vi "Actor Core.vi"(8 "error in":cluster{"状态":bool, "代码":i32, "源":string} caption="错误输入", 11 "JOY in":refnum<class "JoyStick.lvclass">) -> (0 "error out":cluster{"状态":bool, "代码":i32, "源":string} caption="错误输出", 3 "操作者输出":refnum<class "Actor.lvclass">)   [LabVIEW 2014, in "JoyStick.lvlib" / "JoyStick.lvclass"]
doc: "Actor Core.vi包含操作者的主要消息处理循环。操作者通常位于该循环中，在各种消息到达时对消息进行处理。如Do.vi消息返回任何错误，该循环将停止运行，错误代码43将被作为“无错误停止”的标准信号发送给调用方。如需更改上述行为，可在子孙类的Handle Error.vi中对该部分逻辑进行重写。"
uses:
  JoyStick.lvclass
  <vilib>/ActorFramework/Actor/Actor.lvclass
  <vilib>/MakerHub/Xbox-One-Controller/Private/Type Defs/Indicators/All Buttons Visual.ctl
  <vilib>/MakerHub/Xbox-One-Controller/Private/Type Defs/Indicators/A.ctl
  <vilib>/MakerHub/Xbox-One-Controller/Private/Type Defs/Indicators/B.ctl
  <vilib>/MakerHub/Xbox-One-Controller/Private/Type Defs/Indicators/X.ctl
  <vilib>/MakerHub/Xbox-One-Controller/Private/Type Defs/Indicators/Y.ctl
  <vilib>/MakerHub/Xbox-One-Controller/Private/Type Defs/Indicators/Left Bumper.ctl
  <vilib>/MakerHub/Xbox-One-Controller/Private/Type Defs/Indicators/Right Bumper.ctl
  <vilib>/MakerHub/Xbox-One-Controller/Private/Type Defs/Indicators/View.ctl
  <vilib>/MakerHub/Xbox-One-Controller/Private/Type Defs/Indicators/Menu.ctl
  <vilib>/MakerHub/Xbox-One-Controller/Private/Type Defs/Indicators/Thumbstick.ctl
  <vilib>/MakerHub/Xbox-One-Controller/Private/Type Defs/Indicators/All Axis Data.ctl
  <vilib>/MakerHub/Xbox-One-Controller/Private/Type Defs/Indicators/DPad Enum.ctl
  <vilib>/ActorFramework/Actor/Actor.lvclass/Actor.ctl
  JoyStick.lvclass/JoyStick.ctl
  <vilib>/ActorFramework/Message Enqueuer/Message Enqueuer.lvclass/Message Enqueuer.ctl
  <vilib>/ActorFramework/Message Enqueuer/Enqueue.vi
  <vilib>/MakerHub/Xbox-One-Controller/Public/Open First Controller.vi
  <vilib>/ActorFramework/Message Priority Queue/Priority Enqueue.vi
  Wrapper_lib/zsActor/ActorWrapper.lvclass
  <vilib>/MakerHub/Xbox-One-Controller/LMH-Xbox-One-Controller.lvlib
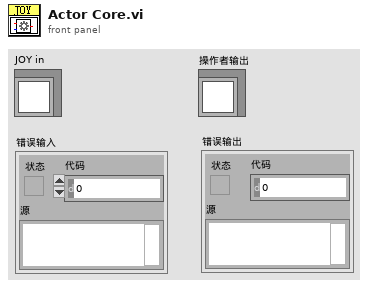
[diagram p1: front panel]
types:
  T1 = typedef "LMH-Xbox-One-Controller.lvlib/All Buttons Visual.ctl" = cluster{"A":T2, "B":T3, "X":T4, "Y":T5, "Left Bumper":T6, "Right Bumper":T7, "View Button":T8, "Menu Button":T9, "Left Stick":T10, "Right Stick":T10}
  T2 = typedef "LMH-Xbox-One-Controller.lvlib/A.ctl" = bool
  T3 = typedef "LMH-Xbox-One-Controller.lvlib/B.ctl" = bool
  T4 = typedef "LMH-Xbox-One-Controller.lvlib/X.ctl" = bool
  T5 = typedef "LMH-Xbox-One-Controller.lvlib/Y.ctl" = bool
  T6 = typedef "LMH-Xbox-One-Controller.lvlib/Left Bumper.ctl" = bool
  T7 = typedef "LMH-Xbox-One-Controller.lvlib/Right Bumper.ctl" = bool
  T8 = typedef "LMH-Xbox-One-Controller.lvlib/View.ctl" = bool
  T9 = typedef "LMH-Xbox-One-Controller.lvlib/Menu.ctl" = bool
  T10 = typedef "LMH-Xbox-One-Controller.lvlib/Thumbstick.ctl" = bool
  T11 = typedef "LMH-Xbox-One-Controller.lvlib/All Axis Data.ctl" = cluster{"Left Stick":cluster{"X Axis":i32, "Y Axis":i32}, "Right Stick":cluster{"X Axis":i32, "Y Axis":i32}, "Triggers":i32, "D-Pad":T12}
  T12 = typedef "LMH-Xbox-One-Controller.lvlib/DPad Enum.ctl" = enum16{"Idle", "Up", "Up / Right", "Right", "Down / Right", "Down", "Down / Left", "Left", "Up / Left"}
  T13 = typedef "LMH-Xbox-One-Controller.lvlib/Xbox One Controller Ref.ctl" = cluster{"Controller Ref":refnum<k1>, "Event Refnum":refnum<event-registration>, "Worker Ref":refnum<vi>}
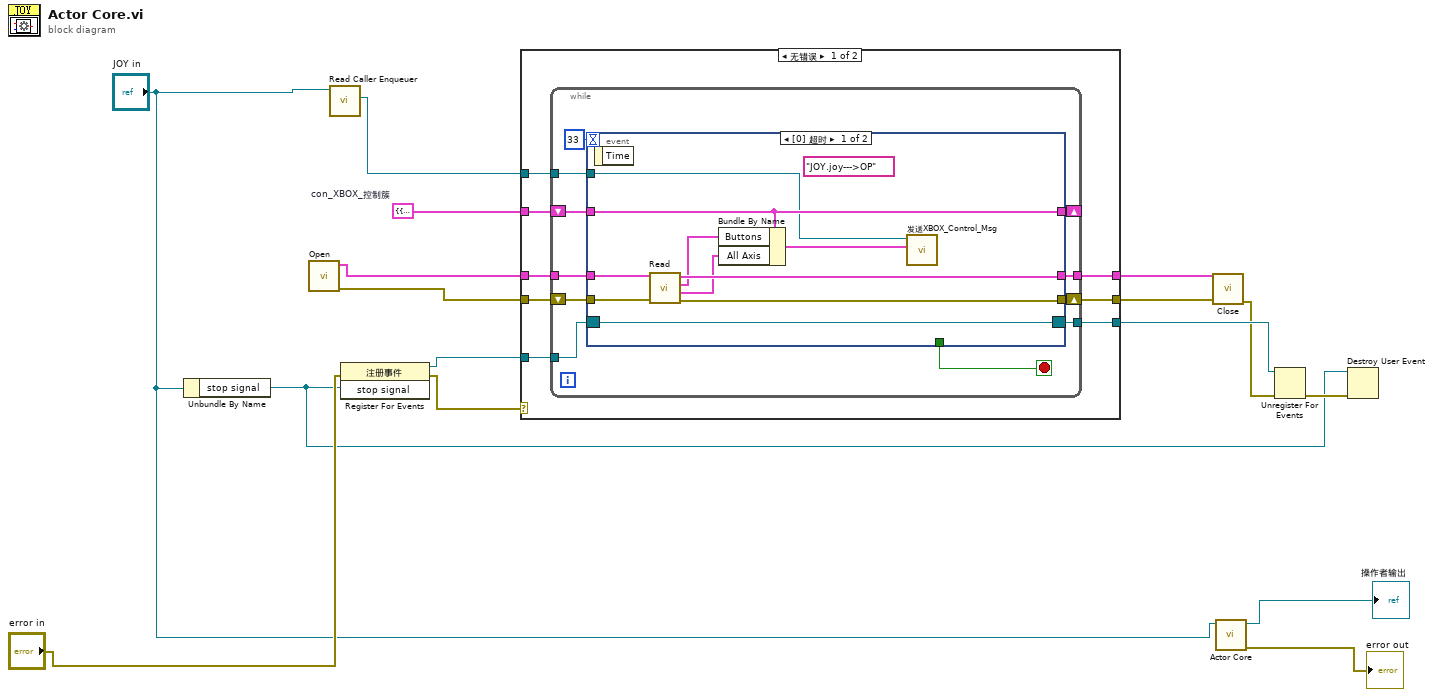
[diagram p0: block diagram]
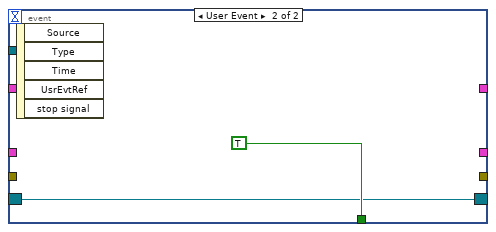
[diagram p2: hidden frame]
diagram:
  w10 = cluster{"Buttons":T1, "All Axis":T11} {"Buttons"={"A"=FALSE, "B"=FALSE, "X"=FALSE, "Y"=FALSE, "Left Bumper"=FALSE, "Right Bumper"=FALSE, "View Button"=FALSE, "Menu Button"=FALSE, "Left Stick"=FALSE, "Right Stick"=FALSE}, "All Axis"={"Left Stick"={"X Axis"=0, "Y Axis"=0}, "Right Stick"={"X Axis"=0, "Y Axis"=0}, "Triggers"=0, "D-Pad"=enum."Idle"}}  # con_XBOX_控制簇
  n1 = Unbundle By Name("JOY in") -> ("stop signal"=w1:refnum<user-event>)
  n2 = call-poly <vilib>:"Open.vi"() -> ("Error Out"=w12:errorcluster, "Xbox One Controller"=w11:T13)  [unwired: 9 in, 1 out]
  n3 = call <vilib>:"Read Caller Enqueuer.vi"("Actor"="JOY in") -> ("Caller Enqueuer"=w9:refnum<class "Message Enqueuer.lvclass">)  [unwired: 10 in]
  n4 = register-events(error in="error in", w1) -> (reference out=w6:refnum<event-registration>, error out=w8:errorcluster)  [unwired: 1 in]
  n5 = case shown="无错误" w8 {
    tunnel: [w24 w50] -> w14
    tunnel: [w23 w49] -> w13
    tunnel: w12 -> [w22 w49]
    tunnel: w11 -> [w21 w50]
    tunnel: w10 -> [w20 _]
    tunnel: w9 -> [w19 _]
    tunnel: w6 -> [w18 w48]
    tunnel: [w17 w48] -> w5
    frame No Error {
      n6 = while {
        shift-right: [w31] -> w23
        shift-left: w22 -> [w34]
        tunnel: w21 -> [w35]
        tunnel: [w33] -> w24
        tunnel: w19 -> [w29]
        shift-right: [w28] -> _
        shift-left: w20 -> [w30]
        tunnel: w18 -> [w27]
        tunnel: [w25] -> w17
        stop <- w26 stop-if-true
        n7 = event shown="[0] 超时" {
          selector: w27 -> [w38 w46]
          dyn-events: [w38 w46] -> w25
          timeout: 33 -> [_ _]
          tunnel: w35 -> [w45 _]
          tunnel: w34 -> [w44 _]
          tunnel: [w43 _] -> w31
          tunnel: [w42 _] -> w33
          tunnel: w30 -> [w41 _]
          tunnel: w29 -> [w36 _]
          tunnel: [w41 _] -> w28
          tunnel: [_ TRUE] -> w26
          event Timeout {
            (unwired) "JOY.joy--->OP" ("Event Text")
            n8 = event-data() -> ()  [unwired: 1 in, 1 out]
            n9 = call <vilib>:"Read.vi"("Error In"=w44, "Xbox One Controller Ref"=w45) -> ("Error Out"=w43:errorcluster, "All Axis"=w39:T11, "Buttons"=w40:T1, "Xbox One Controller Ref"=w42:T13)  [unwired: 6 in]
            n10 = Bundle By Name(cluster=w41, "Buttons"=w40, "All Axis"=w39) -> (w37:cluster{"Buttons":T1, "All Axis":T11})
            n11 = call "发送XBOX_Control_Msg.vi"("XBOX_Control"=w37, "消息待入队列"=w36) -> ()  [unwired: 8 in, 2 out]
          }
          event User Event {
            n12 = event-data() -> ()  [unwired: 1 in, 5 out]
          }
        }
      }
    }
    frame Error {
    }
  }
  n13 = call <vilib>:"Close.vi"("Error In"=w13, "Xbox One Controller Ref"=w14) -> ("Error Out"=w4:errorcluster)  [unwired: 9 in]
  n14 = call-parent "Actor Core.vi"("Actor in"="JOY in") -> ("error out"=→"error out":errorcluster, "Actor out"=→"操作者输出":refnum<class "Actor.lvclass">)  [unwired: 9 in]
  n15 = Unregister For Events(event registration refnum=w5, error in=w4) -> (error out=w7:errorcluster)
  n16 = Destroy User Event(user event=w1, error in=w7) -> ()  [unwired: 1 out]
